vi "fin results.vi"() -> ()   [LabVIEW 2016]
uses:
  <vilib>/Utility/miscctls.llb/LVPoint32TypeDef.ctl
  <vilib>/Utility/miscctls.llb/LVRowAndColumnTypeDef.ctl
  <vilib>/addons/database/Connection.llb/DB Tools Open Connec (String).vi
  <vilib>/addons/database/Connection.llb/Conn Execute.vi
  <vilib>/addons/database/Recordset.llb/Rec Fetch Recordset Data (R).vi
  <vilib>/addons/database/Recordset.llb/Rec Destroy - Connection.vi
  <vilib>/addons/database/NI_Database_API.lvlib
panel:
  out "Cell Position":T1
  out "Coords":T2
  out "seq std":dbl[][](array[numeric])
  out "size(s)":i32[](array[numeric])
  out "element 2":i32
  out "recordset data":variant[][](array[variant])
  out "error out":errorcluster
  out "ItemTag":string
  out "element":string
  out "Item Names":string[](array[string])
  out "PlatMods":T3
  out "Time":u32
  out "Data":T4(array[cluster])
  in  "Listbox":i32[](listbox)=[1]
  in  "stop":bool
  in  "Multicolumn Listbox":i32(listbox)
  out "Array 9":dbl[][][](array[numeric])
  out "Waveform Graph":dbl[](graph)
  in  "length":i32=1
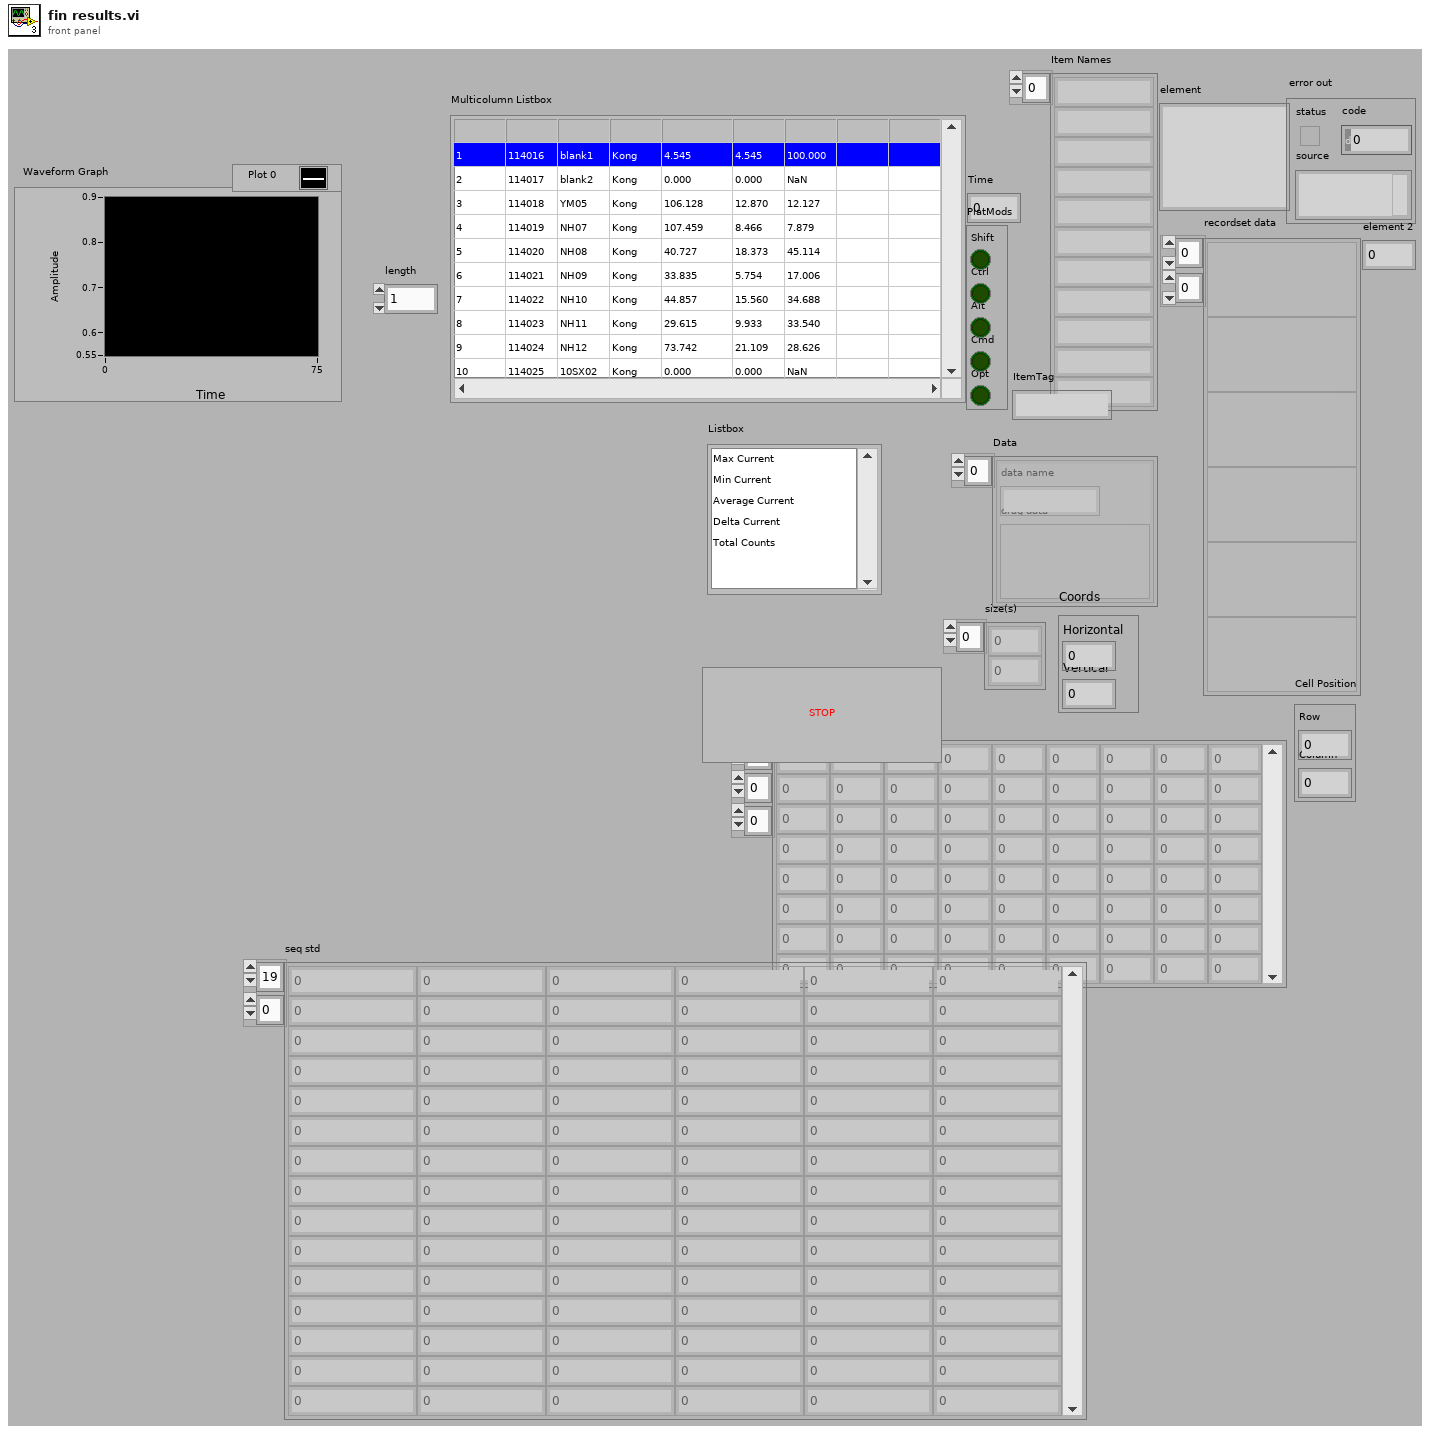
[diagram p1: front panel]
types:
  T1 = typedef "LVRowAndColumnTypeDef.ctl" = cluster{"Row":i32, "Column":i32}
  T2 = typedef "LVPoint32TypeDef.ctl" = cluster{"Horizontal":i32, "Vertical":i32}
  T3 = cluster{"Shift":bool, "Ctrl":bool, "Alt":bool, "Cmd":bool, "Opt":bool}
  T4 = cluster{"data name":string, "drag data":variant}[]
  T5 = typedef "NI_Database_API.lvlib/Conn ObjectReference.ctl" = refnum<k1>
  T6 = typedef "NI_Database_API.lvlib/Rec ObjectReference.ctl" = refnum<k1>
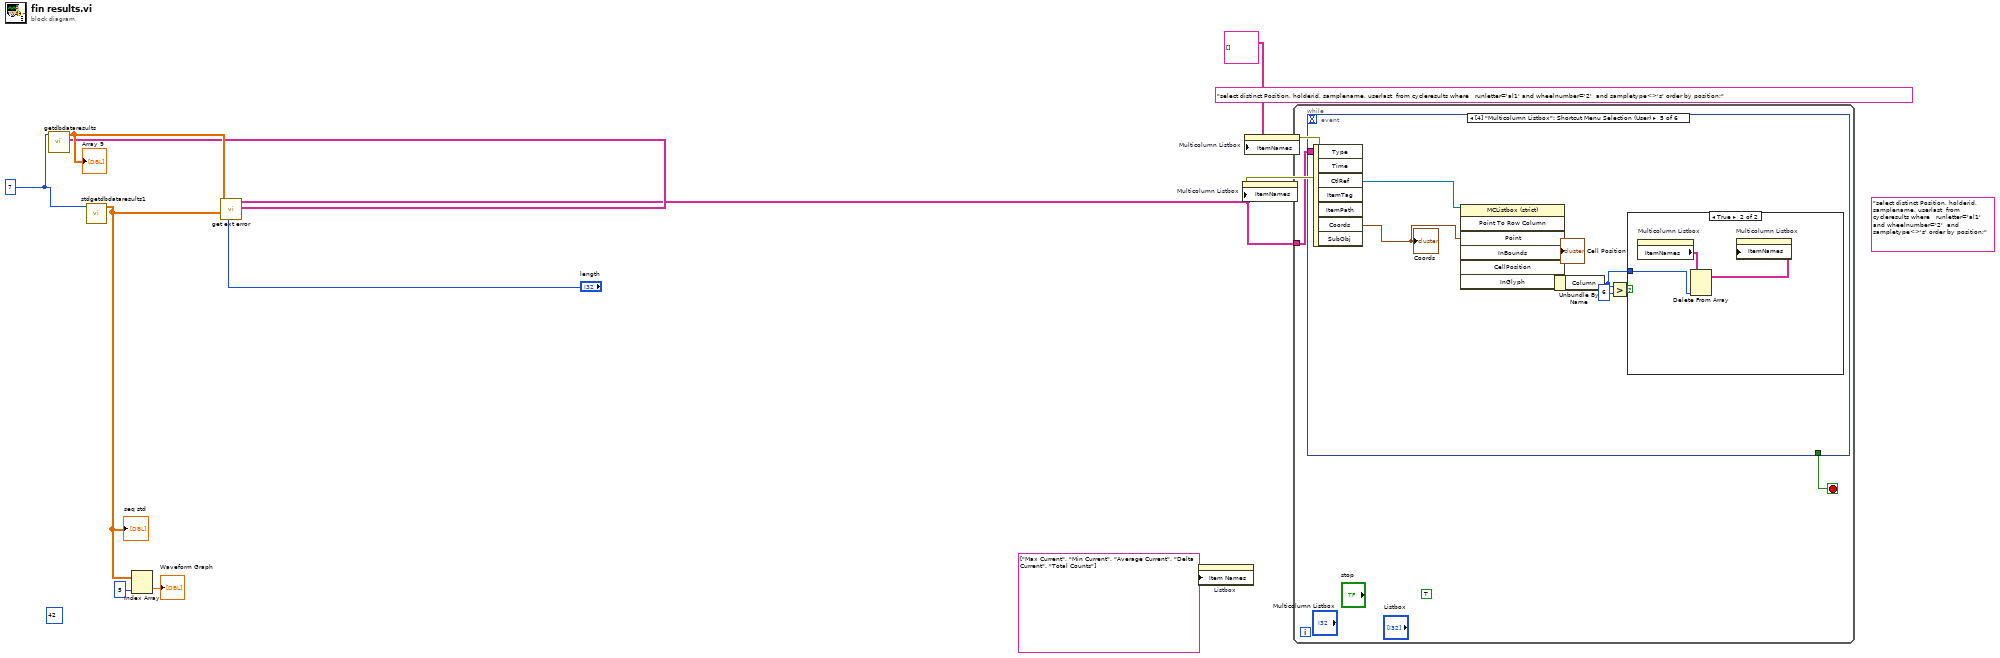
[diagram p0: block diagram]
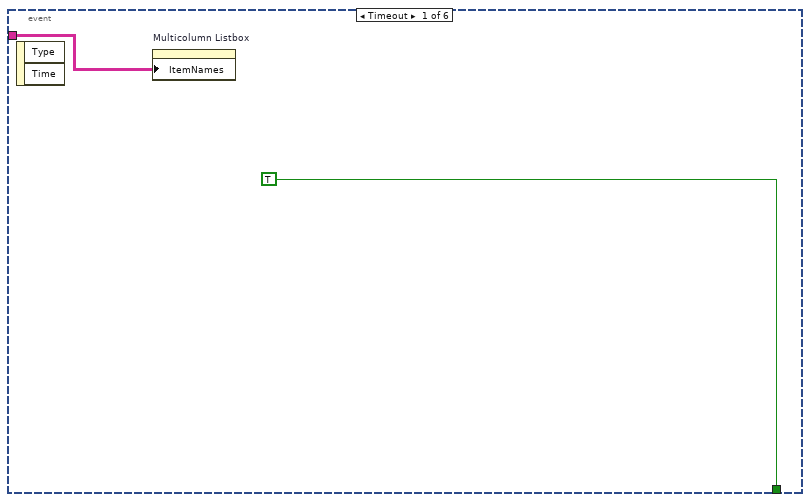
[diagram p2: hidden frame]
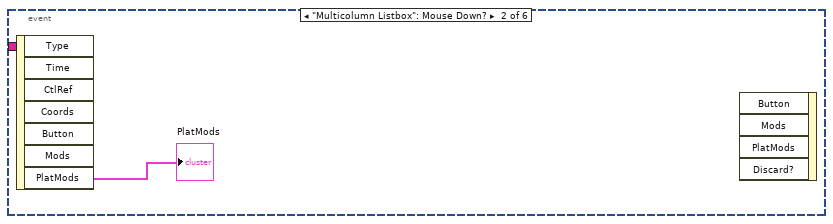
[diagram p3: hidden frame]
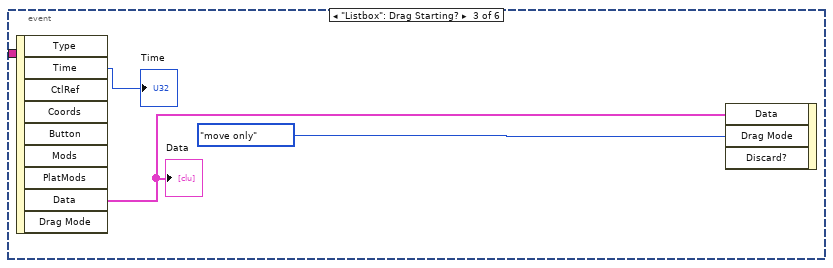
[diagram p4: hidden frame]
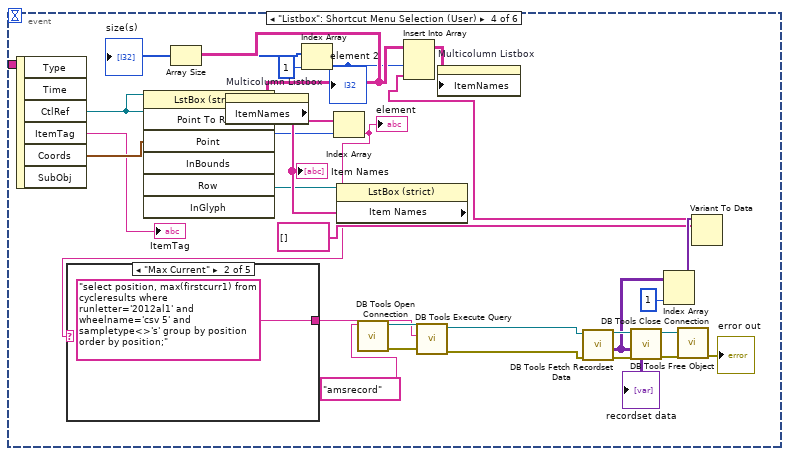
[diagram p5: hidden frame]
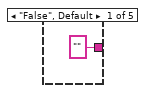
[diagram p6: hidden frame]
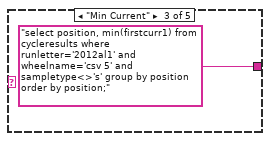
[diagram p7: hidden frame]
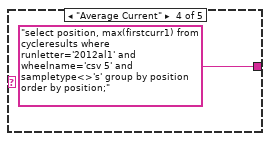
[diagram p8: hidden frame]
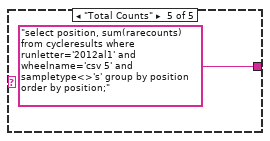
[diagram p9: hidden frame]
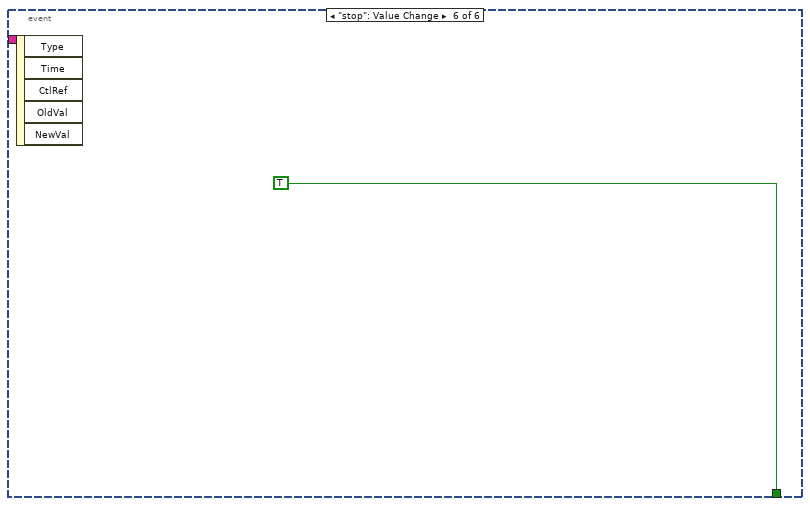
[diagram p11: hidden frame]
diagram:
  w2 = 7 ("charge state")
  (unwired) "select distinct Position, holderid, samplename, userlast  from cycleresults where   runletter='al1' and wheelnumber='2'  and sampletype<>'s' order by position;" ("SQL query get data name")
  (unwired) "select distinct Position, holderid, samplename, userlast  from cycleresults where   runletter='al1' and wheelnumber='2'  and sampletype<>'s' order by position;" ("SQL query")
  (unwired) 42
  n1 = call "getdbdataresults.vi"("charge state"=w2) -> ("sample data"=w10:string[][], "Array 2"=w11:dbl[][][])  [unwired: 6 in, 3 out]
  "Array 9" <- w11
  n2 = call "stdgetdbdataresults1.vi"("charge state"=w2) -> ("seq std"=w9:dbl[][])  [unwired: 9 in, 1 out]
  "seq std" <- w9
  n3 = Index Array(array=w9, index (col)=5 ("disabled index (col)")) -> (element=→"Waveform Graph":dbl[])  [unwired: 1 in]
  n4 = call "get ext error.vi"("length"="length", "seq std"=w9, "sample data"=w10, "unknown data in"=w11) -> ("Array out"=w4:string[][])  [unwired: 6 in, 1 out]
  n5 = property on="Listbox" class="LstBox (strict)"("Item Names"=string[] ["Max Current", "Min Current", "Average Current", "Delta Current", "Total Counts"]) -> ()  [unwired: 2 in, 2 out]
  n6 = property on="Multicolumn Listbox" class="MCListbox (strict)"("ItemNames"=string[][] [] ("Item Names")) -> (error out=w3:errorcluster)  [unwired: 2 in, 1 out]
  n7 = property on="Multicolumn Listbox" class="MCListbox (strict)"(error in=w3, "ItemNames"=w4) -> ()  [unwired: 1 in, 2 out]
  n8 = while {
    tunnel: w4 -> [w13]
    stop <- w12 stop-if-true
    (unwired) TRUE
    n9 = event shown="[4] \"Multicolumn Listbox\": Shortcut Menu Selection (User)" {
      selector: _ -> [_ _ _ _ _ _]
      dyn-events: _ -> [_ _ _ _ _ _]
      timeout: _ -> [_ _ _ _ _ _]
      tunnel: w13 -> [w15 _ _ _ _ _]
      tunnel: [TRUE _ _ _ _ TRUE] -> w12
      event Timeout {
        n10 = event-data() -> ()  [unwired: 1 in, 2 out]
        n11 = property on="Multicolumn Listbox" class="MCListbox (strict)"("ItemNames"=w15) -> ()  [unwired: 2 in, 2 out]
      }
      event "Multicolumn Listbox": Mouse Down? {
        n12 = event-data() -> ("PlatMods"=→"PlatMods":T3)  [unwired: 1 in, 6 out]
        n13 = event-data() -> ()  [unwired: 5 in, 1 out]
      }
      event "Listbox": Drag Starting? {
        n14 = event-data() -> ("Time"=→"Time":u32, "Data"=w18:T4)  [unwired: 1 in, 7 out]
        "Data" <- w18
        n15 = event-data("Data"=w18, "Drag Mode"=enum32{"copy or move", "copy only", "move only"}."move only") -> ()  [unwired: 2 in, 1 out]
      }
      event "Listbox": Shortcut Menu Selection (User) {
        n16 = event-data() -> ("CtlRef"=w43:refnum<vi>, "ItemTag"=→"ItemTag":string, "Coords"=w45:T2)  [unwired: 1 in, 3 out]
        n17 = invoke class="LstBox (strict)" method="Point To Row"(reference=w43, "Point"=w45) -> ("Row"=w44:i32)  [unwired: 5 in, 6 out]
        n18 = property on="Multicolumn Listbox" class="MCListbox (strict)"() -> ("ItemNames"=w26:string[][])  [unwired: 2 in, 2 out]
        n19 = Array Size(array=w26) -> (size(s)=w25:i32[])
        "size(s)" <- w25
        n20 = Index Array(array=w25, index=1) -> (element=w22:i32)
        "element 2" <- w22
        n21 = property class="LstBox (strict)"(reference=w43) -> ("Item Names"=w46:string[])  [unwired: 1 in, 2 out]
        "Item Names" <- w46
        n22 = Index Array(array=w46, index=w44) -> (element=w20:string)
        "element" <- w20
        n23 = case shown="\"Max Current\"" w20 {
          tunnel: ["" ("SQL query") "select position, max(firstcurr1) from cycleresults where runletter='2012al1' and wheelname='csv 5' and sampletype<>'s' group by position order by position;" ("SQL query") "select position, min(firstcurr1) from cycleresults where runletter='2012al1' and wheelname='csv 5' and sampletype<>'s' group by position order by position;" ("SQL query") "select position, max(firstcurr1) from cycleresults where runletter='2012al1' and wheelname='csv 5' and sampletype<>'s' group by position order by position;" ("SQL query") "select position, sum(rarecounts) from cycleresults where runletter='2012al1' and wheelname='csv 5' and sampletype<>'s' group by position order by position;" ("SQL query")] -> w40
          frame "False", Default {
          }
          frame "Max Current" {
          }
          frame "Min Current" {
          }
          frame "Average Current" {
          }
          frame "Total Counts" {
          }
        }
        n24 = call-poly <vilib>:"DB Tools Open Connection.vi"("connection information"="amsrecord" ("password")) -> ("error out"=w42:errorcluster, "connection reference"=w41:T5)  [unwired: 7 in]
        n25 = call-poly <vilib>:"DB Tools Execute Query.vi"("error in (no error)"=w42, "SQL query"=w40, "connection reference"=w41) -> ("error out"=w39:errorcluster, "recordset reference"=w38:T6)  [unwired: 5 in]
        n26 = call-poly <vilib>:"DB Tools Fetch Recordset Data.vi"("error in (no error)"=w39, "recordset reference"=w38) -> ("error out"=w37:errorcluster, "recordset data"=w31:variant[][], "recordset reference out"=w36:T6)  [unwired: 3 in]
        "recordset data" <- w31
        n27 = call-poly <vilib>:"DB Tools Free Object.vi"("error in (no error)"=w37, "recordset reference"=w36) -> ("error out"=w35:errorcluster, "connection reference"=w34:T5)  [unwired: 8 in]
        n28 = Index Array(array=w31, index (col)=1 ("disabled index (col)")) -> (element=w29:variant[])  [unwired: 1 in]
        n29 = call <vilib>:"DB Tools Close Connection.vi"("error in (no error)"=w35, "connection reference"=w34) -> ("error out"=→"error out":errorcluster)  [unwired: 5 in]
        n30 = Variant To Data(type=string[] [], Variant=w29) -> (data=w27:string[])  [unwired: 1 in, 1 out]
        n31 = Insert Into Array(array=w26, index (col)=w22, new element=w27) -> (w23:string[][])  [unwired: 1 in]
        n32 = property on="Multicolumn Listbox" class="MCListbox (strict)"("ItemNames"=w23) -> ()  [unwired: 2 in, 2 out]
      }
      event "Multicolumn Listbox": Shortcut Menu Selection (User) {
        n33 = event-data() -> ("CtlRef"=w57:refnum<vi>, "Coords"=w56:T2)  [unwired: 1 in, 5 out]
        "Coords" <- w56
        n34 = invoke class="MCListbox (strict)" method="Point To Row Column"(reference=w57, "Point"=w56) -> ("CellPosition"=w55:T1)  [unwired: 5 in, 6 out]
        "Cell Position" <- w55
        n35 = Unbundle By Name(w55) -> ("Column"=w52:i32)
        n36 = Greater?(x=w52, y=6) -> (0:w53:bool)
        n37 = case shown="True" w53 {
          tunnel: w52 -> [_ w59]
          frame False {
          }
          frame True {
            n38 = property on="Multicolumn Listbox" class="MCListbox (strict)"() -> ("ItemNames"=w60:string[][])  [unwired: 2 in, 2 out]
            n39 = Delete From Array(array=w60, index (col)=w59) -> (array with subset deleted=w58:string[][])  [unwired: 2 in, 1 out]
            n40 = property on="Multicolumn Listbox" class="MCListbox (strict)"("ItemNames"=w58) -> ()  [unwired: 2 in, 2 out]
          }
        }
      }
      event "stop": Value Change {
        n41 = event-data() -> ()  [unwired: 1 in, 5 out]
      }
    }
  }
